vi "Read.vi"(8 "error in (no error)":errorcluster, 11 "Boolean in":refnum<class "SynchType_SGL.lvclass">) -> (0 "error out":errorcluster, 2 "Value":T1, 3 "Boolean out":refnum<class "SynchType_SGL.lvclass">)   [LabVIEW 2021, in "BT.lvlib" / "SynchType_SGL.lvclass"]
doc: "Abstract Data Classes 2.1.1.12\nTim Streeter - TSA\nCopyright (c) 2024, TSA"
uses:
  SynchType_SGL.lvclass
  SynchType_SGL.lvclass/SynchType_SGL.ctl
  Type.ctl
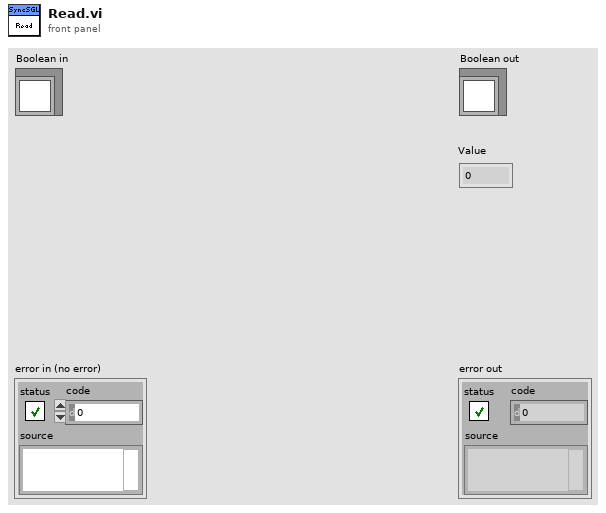
[diagram p1: front panel]
types:
  T1 = typedef "BT.lvlib/SynchType_SGL.lvclass/Type.ctl" = dbl
  T2 = typedef "BT.lvlib/SynchType_DBL.lvclass/Type.ctl" = dbl
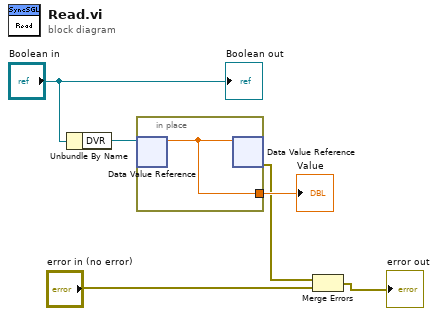
[diagram p0: block diagram]
diagram:
  n1 = Unbundle By Name("Boolean in") -> ("DVR"=w4:refnum<data-value>)
  n2 = in-place {
    in-place-border: [w7] -> w6
    n3 = in-place-dvr #1(w4) -> (w7:T2)  [unwired: 1 out]
    n4 = in-place-dvr #1(w7) -> (w2:errorcluster)  [unwired: 1 out]
  }
  "Value" <- w6
  n5 = Merge Errors(w2, "error in (no error)") -> (→"error out":errorcluster)
  "Boolean out" <- "Boolean in"
